vi "SENS_CORR_CSET_DESC.vi"(0 "VISA IN":refnum<visa-resource-name>, 1 "Calset Description":string, 5 "error in":errorcluster, 7 "Channel":i32) -> (14 "VISA Out":refnum<visa-resource-name>, 19 "error out":errorcluster)   [LabVIEW 2018, in "PNA-X.lvlib"]
doc: "SENSe<cnum>:CORRection:CSET:DESCription <string> \n(Read-Write) Sets or returns the descriptive string assigned to the selected Cal Set. Change this string \nso that you can easily identify each Cal Set. Apply and select the Cal Set using \nSENS:CORR:CSET:ACT. \nParameters \n<cnum> Any existing channel number. If unspecified, value is set to 1 \n<string> The descriptive string associated with the currently-selected Cal Set \nExamples SENS:CORR:CSET:DESC 'MyCalSet' \nsense2:correction:cset:description 'thisCalSet' \nQuery Syntax SENSe<cnum>:CORRection:CSET:DESCription? \nReturn Type String \nDefault Not Applicable"
uses:
  PNA-X.lvlib
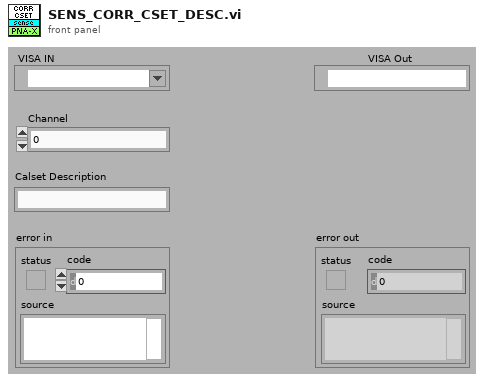
[diagram p1: front panel]
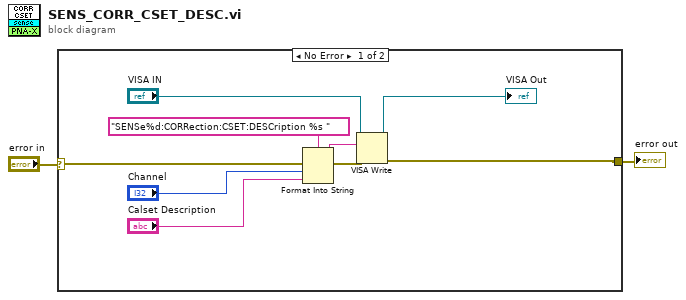
[diagram p0: block diagram]
diagram:
  n1 = case shown="No Error" "error in" {
    selector: "error in" -> [w11 w12]
    tunnel: [w6 w12] -> w1
    frame No Error {
      n2 = Format Into String(format string="SENSe%d:CORRection:CSET:DESCription %s " ("Cmdline"), error in=w11, "Channel", "Calset Description") -> (resulting string=w9:string, error out=w10:errorcluster)  [unwired: 1 in]
      n3 = VISA Write(VISA resource name="VISA IN", write buffer=w9, error in (no error)=w10) -> (VISA resource name out=→"VISA Out":refnum<visa-resource-name>, error out=w6:errorcluster)  [unwired: 1 out]
    }
    frame Error {
    }
  }
  "error out" <- w1
